vi "MakeMatlabExperiment.vi"(8 "error in":errorcluster, 11 "experimentFilepath":path) -> (0 "error out":errorcluster, 1 "erros?":bool, 2 "errors":string, 3 "ExpID":string)   [LabVIEW 2017]
uses:
  Types/ControlValueChangeEventBindingType.ctl
  Types/MatlabBindingDirectionEnum.ctl
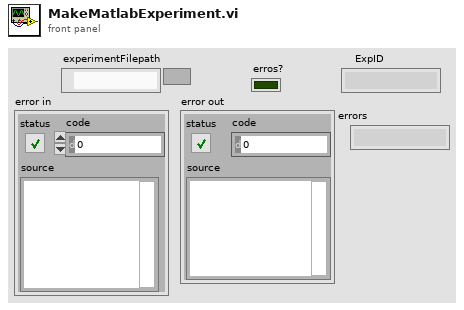
[diagram p1: front panel]
types:
  T1 = typedef "ControlValueChangeEventBindingType.ctl" = cluster{"Control":refnum<vi>, "Event Register":refnum<event-registration>, "AllowVariantValues":bool, "Direction":T2}
  T2 = typedef "MatlabBindingDirectionEnum.ctl" = enum16{"BiDirectional", "FromMatlab", "ToMatlab"}
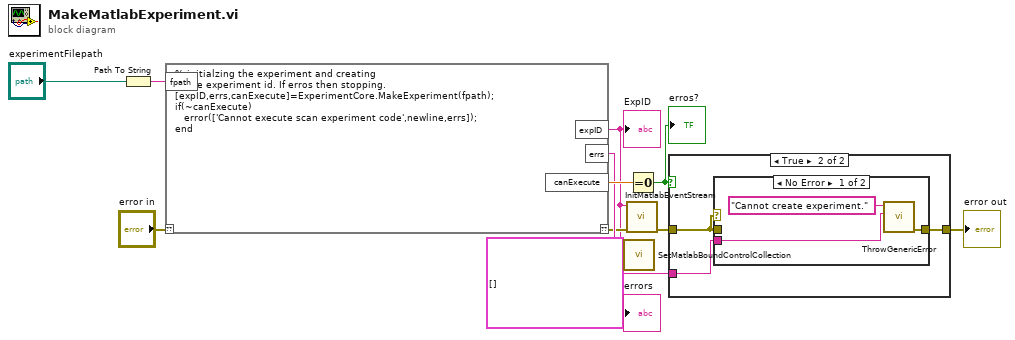
[diagram p0: block diagram]
diagram:
  n1 = Path To String(path="experimentFilepath") -> (string=w11:string)
  n2 = script code="% initialzing the experiment and creating\n% the experiment id. If erros then stopping.\n[expID,errs,canExecute]=ExperimentCore.MakeExperiment(fpath);\nif(~canExecute)\n   error(['Cannot execute scan experiment code',newline,errs]);\nend"("??"="error in", "fpath"=w11) -> ("??"=w3:errorcluster, "expID"=w2:string, "errs"=w6:string, "canExecute"=w9:dbl)
  "ExpID" <- w2
  "errors" <- w6
  n3 = call "SetMatlabBoundControlCollection.vi"("Bound controls"=T1[] [], "ExpID"=w2) -> ()  [unwired: 10 in]
  n4 = call "InitMatlabEventStream.vi"("error in"=w3, "ExpID"=w2) -> ("error out"=w4:errorcluster)  [unwired: 9 in]
  n5 = Equal To 0?(x=w9) -> (x = 0?=w5:bool)
  "erros?" <- w5
  n6 = case shown="True" w5 {
    tunnel: w4 -> [w12 w13]
    tunnel: [w12 w14] -> w7
    tunnel: w6 -> [_ w15]
    frame False {
    }
    frame True {
      n7 = case shown="No Error" w13 {
        tunnel: w13 -> [_ w19]
        tunnel: w15 -> [w17 _]
        tunnel: [w18 w19] -> w14
        frame No Error {
          n8 = call "ThrowGenericError.vi"("Error info"=w17, "TheError"="Cannot create experiment.") -> ("error out"=w18:errorcluster)  [unwired: 9 in]
        }
        frame Error {
        }
      }
    }
  }
  "error out" <- w7
